vi "gestionrh.vi"() -> ()   [LabVIEW 2024]
uses:
  <vilib>/drjdpowell/SQLite Library/SQL Connection/Open (string).vi
  <vilib>/drjdpowell/SQLite Library/SQL Connection/Execute SQL.vi
  <vilib>/drjdpowell/SQLite Library/SQL Connection/Connection.lvclass
  <vilib>/drjdpowell/SQLite Library/SQLite.lvlib
panel:
  in  "Fichier DB":string
  out "Données users":string[][](table) caption="Données user"
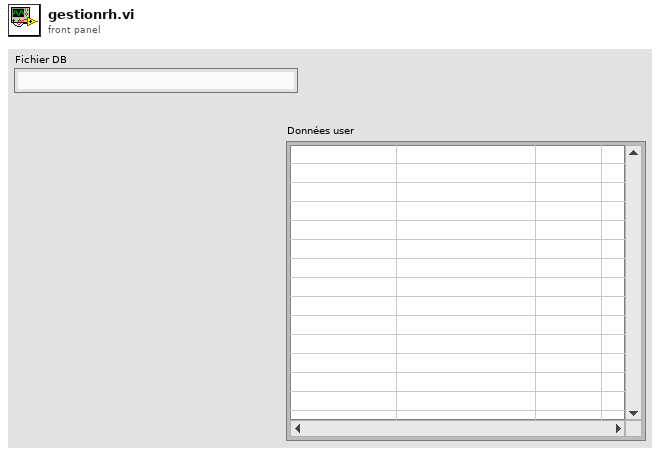
[diagram p1: front panel]
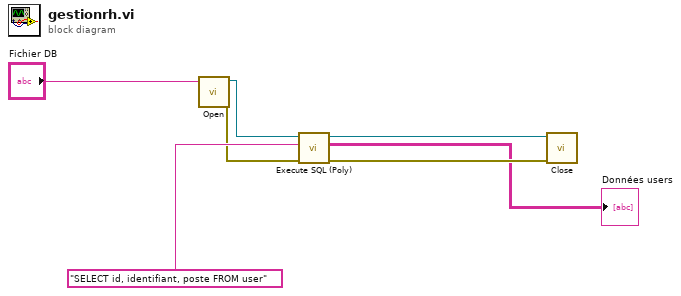
[diagram p0: block diagram]
diagram:
  n1 = call-poly <vilib>:"Open.vi"("db file"="Fichier DB") -> ("error out"=w2:errorcluster, "SQLite Connection"=w3:refnum<class "Connection.lvclass">)  [unwired: 9 in]
  n2 = call-poly <vilib>:"Execute SQL (Poly).vi"("error in (no error)"=w2, "SQL"="SELECT id, identifiant, poste FROM user", "SQLite Connection in"=w3) -> ("error out"=w6:errorcluster, "Result Set"=→"Données users":string[][], "SQLite Connection"=w7:refnum<class "Connection.lvclass">)  [unwired: 5 in, 1 out]
  n3 = call-dynamic "Close.vi"("error in (no error)"=w6, "SQLite Connection in"=w7) -> ()  [unwired: 9 in, 1 out]
